vi "GetComponentGUID.vi"(8 "error in (no error)":errorcluster, 11 "ViPER_Base in":refnum<class "ViPER.lvclass">) -> (0 "error out":errorcluster, 1 "UUID":string, 2 "Version":string, 3 "ViPER_Base out":refnum<class "ViPER.lvclass">)   [LabVIEW 2017]
doc: "### BSD License (http://www.opensource.org/licenses/bsd-license.php) Begin ###\n\nCopyright (c) 2018 Kurt Friday www.medulla.net\n\nAll rights reserved.\n\nRedistribution and use in source and binary forms, with or without\nmodification, are permitted provided that the following conditions are met:\n\n * Redistributions of source code must retain the above copyright\n notice, this list of conditions and the following disclaimer.\n\n * Redistributions in binary form must reproduce the above copyright\n notice, this list of conditions and the following disclaimer in the\n documentation and/or other materials provided with the distribution.\n\n * Neither the name of the <organization> nor the\n names of its contributors may be used to endorse or promote products\n derived from this software without specific prior written permission.\n\nTHIS SOFTWARE IS PROVIDED BY THE COPYRIGHT HOLDERS AND CONTRIBUTORS \"AS IS\" AND\nANY EXPRESS OR IMPLIED WARRANTIES, INCLUDING, BUT NOT LIMITED TO, THE IMPLIED\nWARRANTIES OF MERCHANTABILITY AND FITNESS FOR A PARTICULAR PURPOSE ARE\nDISCLAIMED. IN NO EVENT SHALL <COPYRIGHT HOLDER> BE LIABLE FOR ANY\nDIRECT, INDIRECT, INCIDENTAL, SPECIAL, EXEMPLARY, OR CONSEQUENTIAL DAMAGES\n(INCLUDING, BUT NOT LIMITED TO, PROCUREMENT OF SUBSTITUTE GOODS OR SERVICES;\nLOSS OF USE, DATA, OR PROFITS; OR BUSINESS INTERRUPTION) HOWEVER CAUSED AND\nON ANY THEORY OF LIABILITY, WHETHER IN CONTRACT, STRICT LIABILITY, OR TORT\n(INCLUDING NEGLIGENCE OR OTHERWISE) ARISING IN ANY WAY OUT OF THE USE OF THIS\nSOFTWARE, EVEN IF ADVISED OF THE POSSIBILITY OF SUCH DAMAGE."
uses:
  ViPER.lvclass
panel:
  out "Chain":string
  # "### BSD License (http://www.opensource.org/licenses/bsd-license.php) Begin ###\n\nCopyright (c) 2018  Kurt Friday www.medulla.net\n\nAll rights reserved.\n\nRedistribution and use in source and binary forms, with or without\nmodification, are permitted provided that the following conditions are met:\n\n    * Redistributions of source code must retain the above copyright\n      notice, this list of conditions and the following disclaimer.\n\n    * Redistributions in binary form must reproduce the above copyright\n      notice, this list of conditions and the following disclaimer in the\n      documentation and/or other materials provided with the distribution.\n\n    * Neither the name of the <organization> nor the\n      names of its contributors may be used to endorse or promote products\n      derived from this software without specific prior written permission.\n\nTHIS SOFTWARE IS PROVIDED BY THE COPYRIGHT HOLDERS AND CONTRIBUTORS \"AS IS\" AND\nANY EXPRESS OR IMPLIED WARRANTIES, INCLUDING, BUT NOT LIMITED TO, THE IMPLIED\nWARRANTIES OF MERCHANTABILITY AND FITNESS FOR A PARTICULAR PURPOSE ARE\nDISCLAIMED. IN NO EVENT SHALL <COPYRIGHT HOLDER> BE LIABLE FOR ANY\nDIRECT, INDIRECT, INCIDENTAL, SPECIAL, EXEMPLARY, OR CONSEQUENTIAL DAMAGES\n(INCLUDING, BUT NOT LIMITED TO, PROCUREMENT OF SUBSTITUTE GOODS OR SERVICES;\nLOSS OF USE, DATA, OR PROFITS; OR BUSINESS INTERRUPTION) HOWEVER CAUSED AND\nON ANY THEORY OF LIABILITY, WHETHER IN CONTRACT, STRICT LIABILITY, OR TORT\n(INCLUDING NEGLIGENCE OR OTHERWISE) ARISING IN ANY WAY OUT OF THE USE OF THIS\nSOFTWARE, EVEN IF ADVISED OF THE POSSIBILITY OF SUCH DAMAGE."
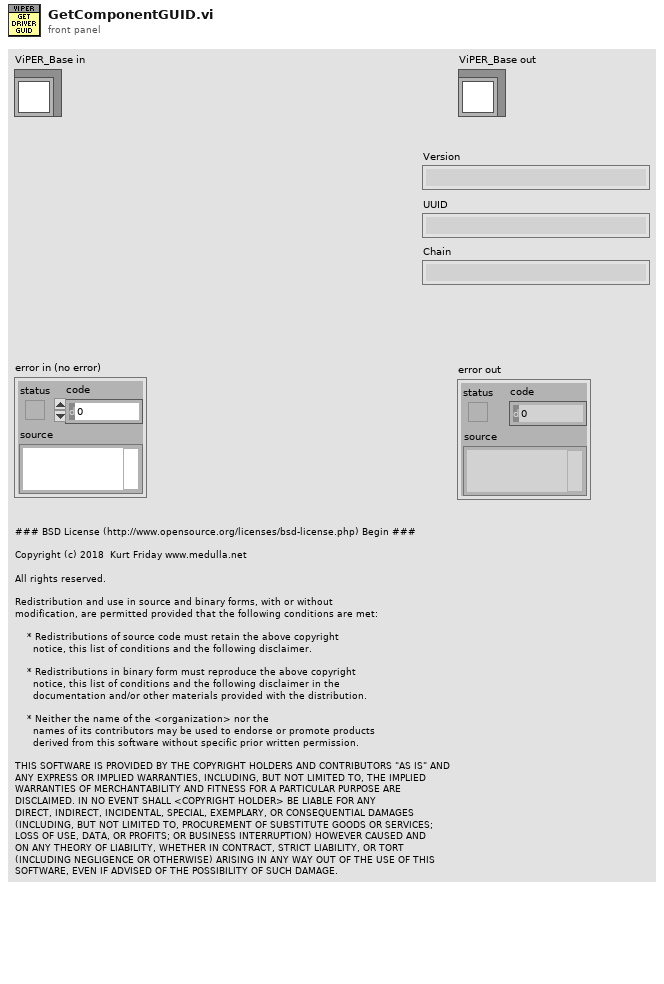
[diagram p1: front panel]
types:
  T1 = cluster{"Major":u16, "Minor":u16, "Fix":u16, "Build":u16}
  T2 = typedef "ViPER.lvlib/ViPER.lvclass/Details.ctl" = cluster{"Name":string, "Class":string}
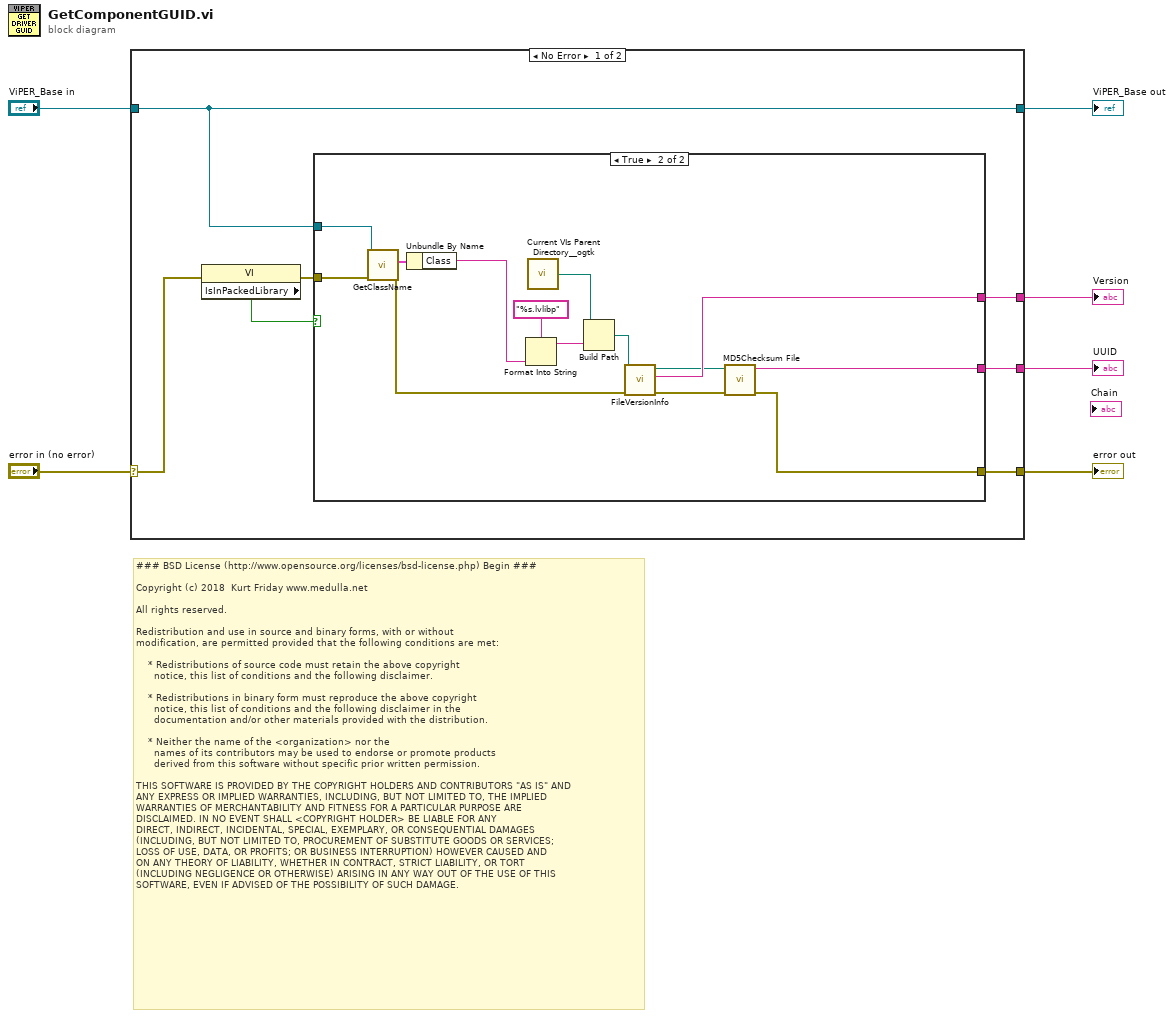
[diagram p0: block diagram]
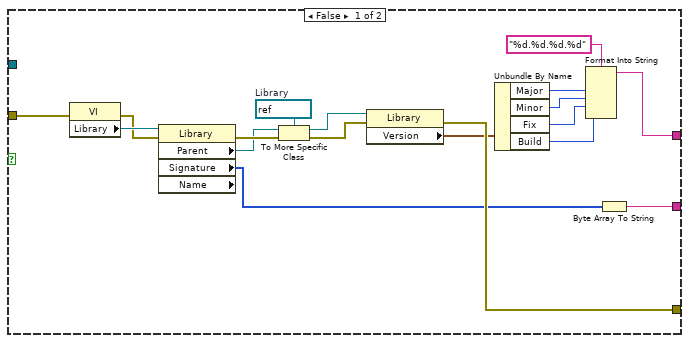
[diagram p2: hidden frame]
diagram:
  # "### BSD License (http://www.opensource.org/licenses/bsd-license.php) Begin ###\n\nCopyright (c) 2018  Kurt Friday www.medulla.net\n\nAll rights reserved.\n\nRedistribution and use in source and binary forms, with or without\nmodification, are permitted provided that the following conditions are met:\n\n    * Redistributions of source code must retain the above copyright\n      notice, this list of conditions and the following disclaimer.\n\n    * Redistributions in binary form must reproduce the above copyright\n      notice, this list of conditions and the following disclaimer in the\n      documentation and/or other materials provided with the distribution.\n\n    * Neither the name of the <organization> nor the\n      names of its contributors may be used to endorse or promote products\n      derived from this software without specific prior written permission.\n\nTHIS SOFTWARE IS PROVIDED BY THE COPYRIGHT HOLDERS AND CONTRIBUTORS \"AS IS\" AND\nANY EXPRESS OR IMPLIED WARRANTIES, INCLUDING, BUT NOT LIMITED TO, THE IMPLIED\nWARRANTIES OF MERCHANTABILITY AND FITNESS FOR A PARTICULAR PURPOSE ARE\nDISCLAIMED. IN NO EVENT SHALL <COPYRIGHT HOLDER> BE LIABLE FOR ANY\nDIRECT, INDIRECT, INCIDENTAL, SPECIAL, EXEMPLARY, OR CONSEQUENTIAL DAMAGES\n(INCLUDING, BUT NOT LIMITED TO, PROCUREMENT OF SUBSTITUTE GOODS OR SERVICES;\nLOSS OF USE, DATA, OR PROFITS; OR BUSINESS INTERRUPTION) HOWEVER CAUSED AND\nON ANY THEORY OF LIABILITY, WHETHER IN CONTRACT, STRICT LIABILITY, OR TORT\n(INCLUDING NEGLIGENCE OR OTHERWISE) ARISING IN ANY WAY OUT OF THE USE OF THIS\nSOFTWARE, EVEN IF ADVISED OF THE POSSIBILITY OF SUCH DAMAGE."
  n1 = case shown="No Error" "error in (no error)" {
    selector: "error in (no error)" -> [w13 w47]
    tunnel: [w11 w47] -> w5
    tunnel: [w12 w46] -> w3
    tunnel: "ViPER_Base in" -> [w12 w46]
    tunnel: [w9 _] -> w2
    tunnel: [w10 _] -> w1
    frame No Error {
      n2 = property class="VI"(error in=w13) -> (error out=w8:errorcluster, "IsInPackedLibrary"=w7:bool)  [unwired: 1 in, 1 out]
      n3 = case shown="True" w7 {
        tunnel: [w14 w37] -> w10
        tunnel: [w28 w36] -> w11
        tunnel: w8 -> [w23 w38]
        tunnel: w12 -> [_ w39]
        tunnel: [w15 w34] -> w9
        frame False {
          w29 = refnum<vi> refnum  # Library
          n4 = property class="VI"(error in=w23) -> (error out=w27:errorcluster, "Library"=w31:refnum<vi>)  [unwired: 1 in, 1 out]
          n5 = property class="Library" props=["Parent", "Signature", "Name"](reference=w31, error in=w27) -> (error out=w30:errorcluster, "Parent"=w26:refnum<vi>, "Signature"=w16:u8[])  [unwired: 2 out]
          n6 = To More Specific Class(target class=w29, reference=w26, error in=w30) -> (specific class reference=w24:refnum<vi>, error out=w25:errorcluster)
          n7 = property class="Library"(reference=w24, error in=w25) -> (error out=w28:errorcluster, "Version"=w22:T1)  [unwired: 1 out]
          n8 = Unbundle By Name(w22) -> ("Major"=w21:u16, "Minor"=w20:u16, "Fix"=w19:u16, "Build"=w18:u16)
          n9 = Format Into String(format string="%d.%d.%d.%d", w21, w20, w19, w18) -> (resulting string=w14:string)  [unwired: 2 in, 1 out]
          n10 = Byte Array To String(unsigned byte array=w16) -> (string=w15:string)
        }
        frame True {
          n11 = call "GetClassName.vi"("error in (no error)"=w38, "reference in"=w39) -> ("error out"=w33:errorcluster, "Details"=w42:T2)  [unwired: 7 in, 1 out]
          n12 = Unbundle By Name(w42) -> ("Class"=w41:string)
          n13 = Format Into String(format string="%s.lvlibp", w41) -> (resulting string=w43:string)  [unwired: 2 in, 1 out]
          n14 = call <userlib>:"Current VIs Parent Directory__ogtk.vi"() -> ("Parent Directory (+ Relative)"=w45:path)  [unwired: 5 in]
          n15 = Build Path(base path=w45, name or relative path=w43) -> (appended path=w40:path)
          n16 = call <vilib>:"FileVersionInfo.vi"("error in (no error)"=w33, "Application Path in"=w40) -> ("error out"=w32:errorcluster, "File Version Info"=w37:string, "Application Path out"=w35:path)  [unwired: 6 in, 1 out]
          n17 = call <vilib>:"MD5Checksum File.vi"("error in (no error)"=w32, "Path"=w35) -> ("error out"=w36:errorcluster, "MD5 message-digest"=w34:string)  [unwired: 8 in]
        }
      }
    }
    frame Error {
    }
  }
  "error out" <- w5
  "ViPER_Base out" <- w3
  "Version" <- w1
  "UUID" <- w2
